vi "golpi_mpc_release.vi"(8 "error in":errorcluster, 10 "golpi ref or golpi session in":variant, 11 "golpi session ref":T1) -> (0 "error out":errorcluster, 3 "golpi session out (copy)":T1)   [LabVIEW 2013, in "GOLPI Multi Process.lvlib"]
doc: "Multi-process GOLPI: call this when you are done with exclusive access GOLPI operations. It releases exclusive access to the GOLPI and stores local copy of GOLPI session or GOLPI ref back to the referenced session.\nIt can accept either GOLPI ref or full GOLPI session as a variant input. Decision which one to assing depneds on user. Typically store just GOLPI ref. Full GOLPI session needs to be stored only if some changes were made in the session."
uses:
  GOLPI Multi Process.lvlib
  golpi_session_ref.ctl
  golpi_session.ctl
  GOLPI Library.lvlibp/Public/GOLPI reference Type Def.ctl
  GOLPI Library.lvlibp/LV Process source distribution/Pipe Handle.ctl
  GOLPI Library.lvlibp/LV Process source distribution/LV Process library.lvlib
  GOLPI Library.lvlibp
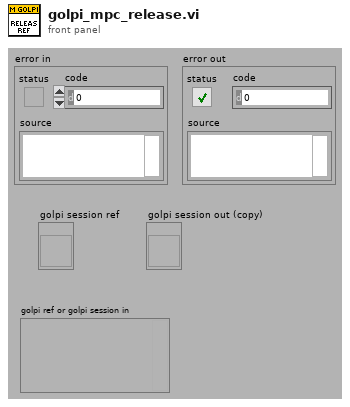
[diagram p1: front panel]
types:
  T1 = typedef "GOLPI Multi Process.lvlib/golpi_session_ref.ctl" = refnum<vi>
  T2 = typedef "GOLPI Library.lvlibp/GOLPI reference Type Def.ctl" = cluster{"pipe handle":T3, "fast read timeout [ms]":u32, "fast read settle time [ms]":u32, "fast read to multiple [ms]":u32, "max elements per input line":u32, "slow read timeout [ms]":u32, "stdin double format specifier":string, "max elements per stdout output column":u32, "console mode bitstream":bool, "bitstream first read timeout [ms]":u32, "bitstream read timeout [ms]":u32, "struct transfer possible":bool, "matlab mode":bool}
  T3 = typedef "GOLPI Library.lvlibp/LV Process library.lvlib/Pipe Handle.ctl" = cluster{"lv_proc.dll file path":path, "process instance handle":u32[], "debug mode":bool, "debug data":cluster{"time":timestamp, "stdin":bool, "data":string}[]}
  T4 = typedef "GOLPI Multi Process.lvlib/golpi_session.ctl" = cluster{"GOLPI ref":T2, "idn str":string, "octave path":path, "work path":path, "start timeout [ms]":u32, "clr cache":bool, "console":bool, "binary":bool, "semaphore":T5, "initial command":string, "exit command":string, "matlab":bool, "pkg list":string[]}
  T5 = typedef "Semaphore RefNum" = refnum<k1>
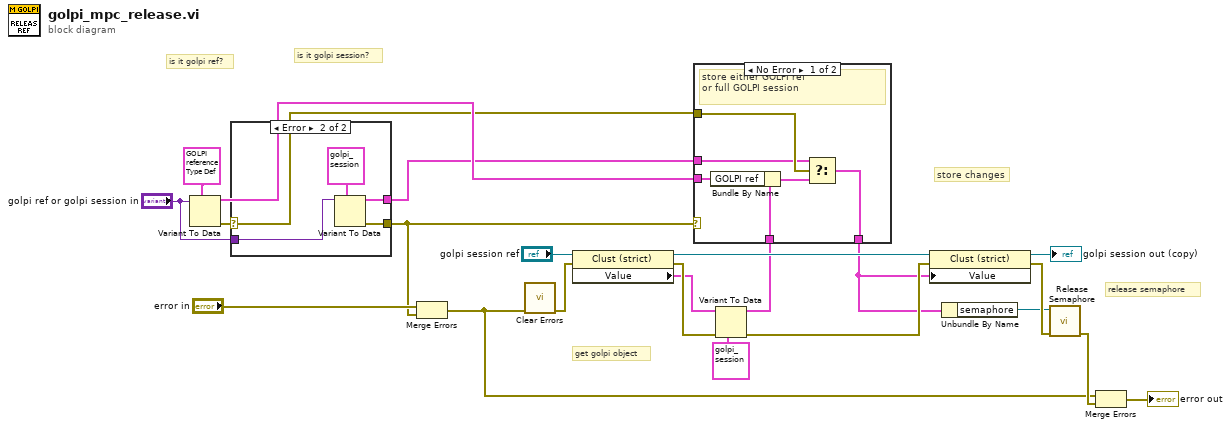
[diagram p0: block diagram]
diagram:
  # "is it golpi session?"
  # "is it golpi ref?"
  # "release semaphore"
  # "store changes"
  # "get golpi object"
  n1 = Variant To Data(type=T2 {"pipe handle"={"lv_proc.dll file path"=path "", "process instance handle"=[], "debug mode"=FALSE, "debug data"=[]}, "fast read timeout [ms]"=0, "fast read settle time [ms]"=0, "fast read to multiple [ms]"=0, "max elements per input line"=0, "slow read timeout [ms]"=0, "stdin double format specifier"="", "max elements per stdout output column"=0, "console mode bitstream"=FALSE, "bitstream first read timeout [ms]"=0, "bitstream read timeout [ms]"=0, "struct transfer possible"=FALSE, "matlab mode"=FALSE} ("golpi ref in"), Variant="golpi ref or golpi session in") -> (data=w4:T2, error out=w3:errorcluster)  [unwired: 1 in]
  n2 = case shown="Error" w3 {
    selector: w3 -> [w23 _]
    tunnel: "golpi ref or golpi session in" -> [_ w26]
    tunnel: [_ w25] -> w2
    tunnel: [w23 w24] -> w5
    frame No Error {
    }
    frame Error {
      n3 = Variant To Data(type=T4 {"GOLPI ref"={"pipe handle"={"lv_proc.dll file path"=path "", "process instance handle"=[], "debug mode"=FALSE, "debug data"=[]}, "fast read timeout [ms]"=0, "fast read settle time [ms]"=0, "fast read to multiple [ms]"=0, "max elements per input line"=0, "slow read timeout [ms]"=0, "stdin double format specifier"="", "max elements per stdout output column"=0, "console mode bitstream"=FALSE, "bitstream first read timeout [ms]"=0, "bitstream read timeout [ms]"=0, "struct transfer possible"=FALSE, "matlab mode"=FALSE}, "idn str"="", "octave path"=path "C:/Octave364/Octave3.6.4_gcc4.6.2/bin", "work path"=path "", "start timeout [ms]"=0, "clr cache"=FALSE, "console"=FALSE, "binary"=FALSE, "semaphore"=refnum, "initial command"="", "exit command"="", "matlab"=FALSE, "pkg list"=[]} ("golpi session in (not used)"), Variant=w26) -> (data=w25:T4, error out=w24:errorcluster)  [unwired: 1 in]
    }
  }
  n4 = Merge Errors("error in", w5) -> (w6:errorcluster)
  n5 = call <vilib>:"Clear Errors.vi"("error in (no error)"=w6) -> ("error out"=w15:errorcluster)  [unwired: 6 in]
  n6 = property class="Clust (strict)"(reference="golpi session ref", error in=w15) -> (reference out=w19:T1, error out=w22:errorcluster, "Value"=w21:T4)
  n7 = Variant To Data(error in=w22, type=T4 {"GOLPI ref"={"pipe handle"={"lv_proc.dll file path"=path "", "process instance handle"=[], "debug mode"=FALSE, "debug data"=[]}, "fast read timeout [ms]"=0, "fast read settle time [ms]"=0, "fast read to multiple [ms]"=0, "max elements per input line"=0, "slow read timeout [ms]"=0, "stdin double format specifier"="", "max elements per stdout output column"=0, "console mode bitstream"=FALSE, "bitstream first read timeout [ms]"=0, "bitstream read timeout [ms]"=0, "struct transfer possible"=FALSE, "matlab mode"=FALSE}, "idn str"="", "octave path"=path "C:/Octave364/Octave3.6.4_gcc4.6.2/bin", "work path"=path "", "start timeout [ms]"=0, "clr cache"=FALSE, "console"=FALSE, "binary"=FALSE, "semaphore"=refnum, "initial command"="", "exit command"="", "matlab"=FALSE, "pkg list"=[]} ("golpi session"), Variant=w21) -> (data=w9:T4, error out=w18:errorcluster)
  n8 = case shown="No Error" w5 {
    tunnel: [w32 w34] -> w1
    tunnel: w9 -> [w33 w34]
    tunnel: w4 -> [w30 _]
    tunnel: w3 -> [w29 _]
    tunnel: w2 -> [w28 _]
    frame No Error {
      # "store either GOLPI ref\nor full GOLPI session"
      n9 = Bundle By Name(cluster=w33, "GOLPI ref"=w30) -> (w31:T4)
      n10 = Select(t=w28, s=w29, f=w31) -> (s? t:f=w32:T4)
    }
    frame Error {
      # "invalid input wired but\nwe must release the semaphore\nanyway otherwise it \nwill lock up forever - \nso return unchanged golpi session"
    }
  }
  n11 = property class="Clust (strict)"(reference=w19, error in=w18, "Value"=w1) -> (reference out=→"golpi session out (copy)":T1, error out=w17:errorcluster)
  n12 = Unbundle By Name(w1) -> ("semaphore"=w16:T5)
  n13 = call <vilib>:"Release Semaphore.vi"("error in (no error)"=w17, "semaphore"=w16) -> ("error out"=w14:errorcluster)  [unwired: 4 in, 1 out]
  n14 = Merge Errors(w6, w14) -> (→"error out":errorcluster)
